vi "Parse 20-1.vi"(11 "String":string) -> (3 "Puzzle":T1)   [LabVIEW 2020]
uses:
  Puzzle 20-1.ctl
  Vec2.ctl
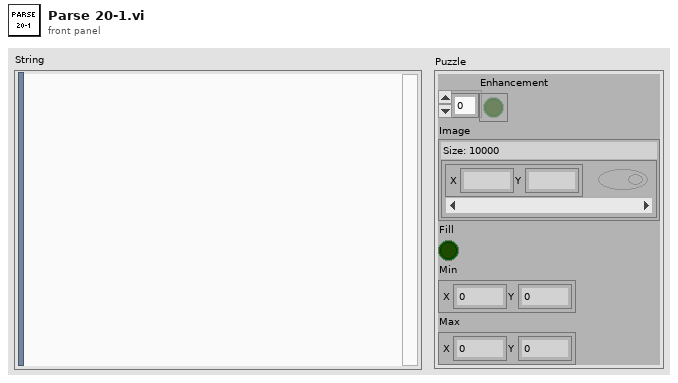
[diagram p1: front panel]
types:
  T1 = typedef "Puzzle 20-1.ctl" = cluster{"Enhancement":bool[], "Image":map{T2, bool}, "Fill":bool, "Min":T2, "Max":T2}
  T2 = typedef "Vec2.ctl" = cluster{"X":i32, "Y":i32}
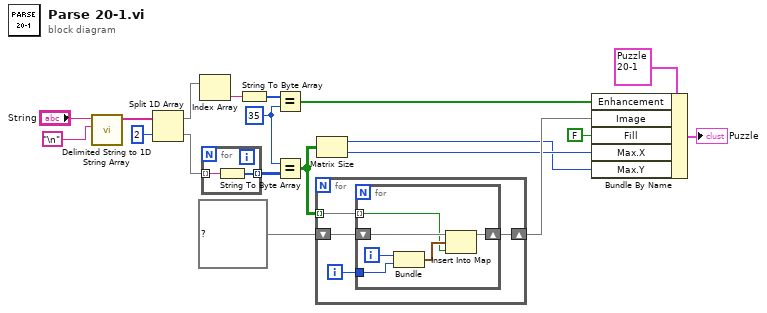
[diagram p0: block diagram]
diagram:
  w8 = u8 35
  n1 = call <vilib>:"Delimited String to 1D String Array.vi"("delimiter"="\n", "delimited string"="String") -> ("string array"=w17:string[])  [unwired: 9 in]
  n2 = Split 1D Array(array=w17, index=2) -> (first subarray=w15:string[], second subarray=w10:string[])
  n3 = Index Array(array=w15) -> (element=w14:string)  [unwired: 1 in]
  n4 = for {
    tunnel: w10 -> [w21] mode=indexing
    tunnel: [w20] -> w9 mode=indexing
    n5 = String To Byte Array(string=w21) -> (unsigned byte array=w20:u8[])
  }
  n6 = String To Byte Array(string=w14) -> (unsigned byte array=w13:u8[])
  n7 = Equal?(x=w13, y=w8) -> (x = y?=w11:bool[])
  n8 = Equal?(x=w8, y=w9) -> (x = y?=w4:bool[][])
  n9 = for {
    tunnel: w4 -> [w25] mode=indexing
    shift-right: [w23] -> w6
    shift-left: map{T2, bool} {} ("Image") -> [w24]
    i -> [w22]
    n10 = for {
      tunnel: w25 -> [w27] mode=indexing
      shift-right: [w26] -> w23
      shift-left: w24 -> [w29]
      tunnel: w22 -> [w30]
      i -> [w31]
      n11 = Bundle(w31, w30) -> (w28:cluster{i32, i32})  [unwired: 1 in]
      n12 = Insert Into Map(map in=w29, key=w28, value=w27) -> (map out=w26:map{T2, bool})  [unwired: 2 out]
    }
  }
  n13 = Matrix Size(0:w4) -> (1:w2:i32, 2:w3:i32)
  n14 = Bundle By Name(cluster=T1 {"Enhancement"=[], "Image"={}, "Fill"=FALSE, "Min"={"X"=0, "Y"=0}, "Max"={"X"=0, "Y"=0}} ("Puzzle 20-1"), "Enhancement"=w11, "Image"=w6, "Fill"=FALSE, "Max.X"=w3, "Max.Y"=w2) -> (→"Puzzle":T1)
